vi "Alignment.vi"() -> ()   [LabVIEW 2010]
uses:
  <vilib>/Utility/inputDevices.llb/closeKeyboard.vi
  <vilib>/Utility/inputDevices.llb/keyboardAcquire.vi
panel:
  out "Q":bool
  out "Further":bool
  out "Nearer":bool
  out "End":bool=TRUE
  out "Right":bool
  out "Up":bool
  out "Left":bool
  out "Down":bool
  in  "Motor GPIB":u8=6 max=32 step=1 format="%#.0f"
  out "keys pressed":T1(array[ring])
  # "Press \"=\" for complete tower down."
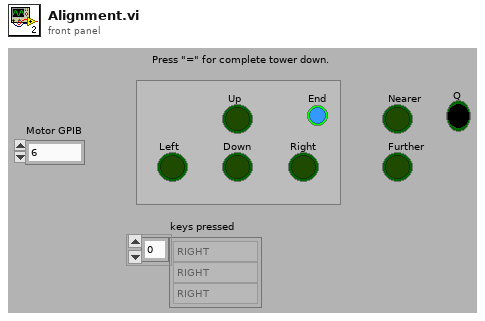
[diagram p1: front panel]
types:
  T1 = enum16{"0", "1", "2", "3", "4", "5", "6", "7", "8", "9", "A", "B", "C", "D", "E", "F", "G", "H", "I", "J", "K", "L", "M", "N", "O", "P", "Q", "R", "S", "T", "U", "V", "W", "X", "Y", "Z", "F1", "F2", "F3", "F4", "F5", "F6", "F7", "F8", "F9", "F10", "F11", "F12", "F13", "F14", "F15", "ADD", "BACK", "BACKSLASH", "CAPITAL", "COMMA", "DECIMAL", "DELETE", "DIVIDE", "DOWN", "END", "EQUALS", "ESCAPE", "GRAVE (`)", "HOME", "INSERT", "LBRACKET", "LCONTROL", "LEFT", "L ALT", "LSHIFT", "LWIN", "MINUS", "MULTIPLY", "NEXT", "NUMLOCK", "NUMPAD_0", "NUMPAD_1", "NUMPAD_2", "NUMPAD_3", "NUMPAD_4", "NUMPAD_5", "NUMPAD_6", "NUMPAD_7", "NUMPAD_8", "NUMPAD_9", "PAUSE", "PERIOD", "PRIOR (PG UP)", "RBRACKET", "RCONTROL", "RETURN", "RIGHT", "R ALT", "RSHIFT", "RWIN", "SCROLL", "SEMICOLON", "SLASH", "SPACE", "SUBTRACT", "TAB", "UP", "ENTER (num pad)", "' (quote)"}[]
  T2 = enum16{"0", "1", "2", "3", "4", "5", "6", "7", "8", "9", "A", "B", "C", "D", "E", "F", "G", "H", "I", "J", "K", "L", "M", "N", "O", "P", "Q", "R", "S", "T", "U", "V", "W", "X", "Y", "Z", "F1", "F2", "F3", "F4", "F5", "F6", "F7", "F8", "F9", "F10", "F11", "F12", "F13", "F14", "F15", "ADD", "BACK", "BACKSLASH", "CAPITAL", "COMMA", "DECIMAL", "DELETE", "DIVIDE", "DOWN", "END", "EQUALS", "ESCAPE", "GRAVE (`)", "HOME", "INSERT", "LBRACKET", "LCONTROL", "LEFT", "L ALT", "LSHIFT", "LWIN", "MINUS", "MULTIPLY", "NEXT", "NUMLOCK", "NUMPAD_0", "NUMPAD_1", "NUMPAD_2", "NUMPAD_3", "NUMPAD_4", "NUMPAD_5", "NUMPAD_6", "NUMPAD_7", "NUMPAD_8", "NUMPAD_9", "PAUSE", "PERIOD", "PRIOR (PG UP)", "RBRACKET", "RCONTROL", "RETURN", "RIGHT", "R ALT", "RSHIFT", "RWIN", "SCROLL", "SEMICOLON", "SLASH", "SPACE", "SUBTRACT", "TAB", "UP", "ENTER (num pad)", "' (quote)"}
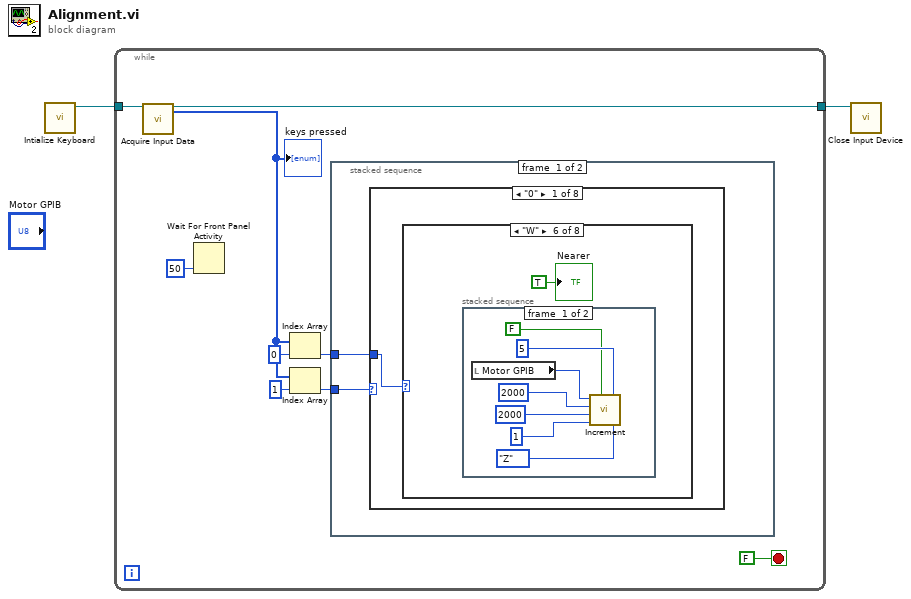
[diagram p0: block diagram]
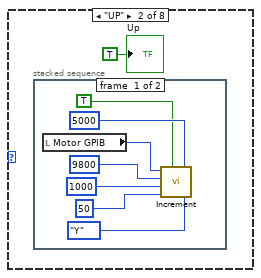
[diagram p3: hidden frame]
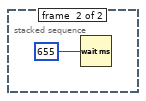
[diagram p4: hidden frame]
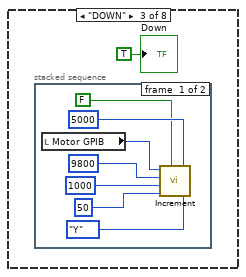
[diagram p5: hidden frame]
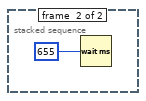
[diagram p6: hidden frame]
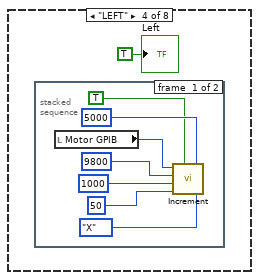
[diagram p7: hidden frame]
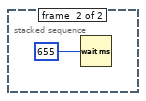
[diagram p8: hidden frame]
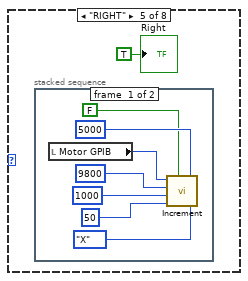
[diagram p9: hidden frame]
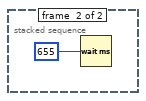
[diagram p10: hidden frame]
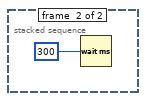
[diagram p11: hidden frame]
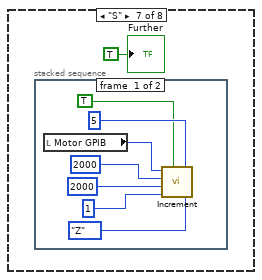
[diagram p12: hidden frame]
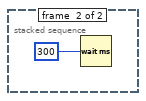
[diagram p13: hidden frame]
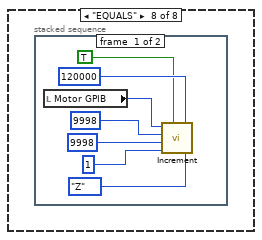
[diagram p14: hidden frame]
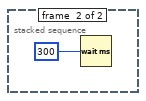
[diagram p15: hidden frame]
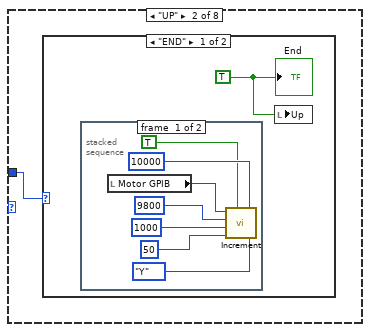
[diagram p16: hidden frame]
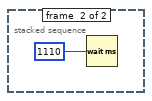
[diagram p17: hidden frame]
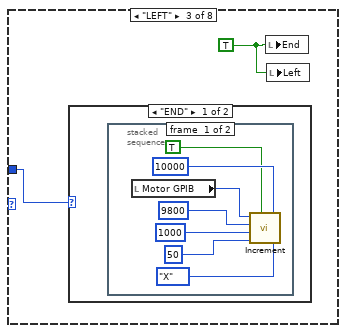
[diagram p19: hidden frame]
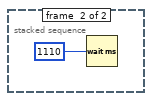
[diagram p20: hidden frame]
diagram:
  n1 = call <vilib>:"Intialize Keyboard.vi"() -> ("device ID"=w1:refnum<k1>)  [unwired: 10 in, 1 out]
  n2 = while {
    tunnel: w1 -> [w11]
    tunnel: [w10] -> w2
    stop <- FALSE stop-if-true
    n3 = call-poly <vilib>:"Acquire Input Data.vi"("device ID"=w11) -> ("device ID"=w10:refnum<k1>, "keys pressed"=w8:T1)  [unwired: 16 in, 1 out]
    "keys pressed" <- w8
    n4 = Wait For Front Panel Activity(1:50 ("timeout ms (-1 never timeout)")) -> ()  [unwired: 2 in, 1 out]
    n5 = Index Array(array=w8, index=0) -> (element=w4:T2)
    n6 = Index Array(array=w8, index=1) -> (element=w5:T2)
    n7 = stacked-sequence {
      tunnel: w5 -> [w13 _]
      tunnel: w4 -> [w12 _]
      frame #0 {
        n8 = case shown="\"0\"" w13 {
          tunnel: w12 -> [w14 w77 w87 w98 w107 w117 w127 _]
          frame "0" {
            n9 = case shown="\"W\"" w14 {
              frame "0", Default {
              }
              frame "UP" {
                n10 = stacked-sequence {
                  frame #0 {
                    n11 = local read "Motor GPIB"() -> (w22:u8)
                    n12 = call "Increment.vi"("GPIB_Addr"=w22, "F Speed"=u16 9800, "L Speed"=u16 1000, "Rate"=u16 50, "CCW 3"=TRUE, "Distance"=u32 5000, "Axis"=enum16{"X", "Y", "Z", "U", "V", "W"}."Y") -> ()
                  }
                  frame #1 {
                    n13 = Wait (ms)(milliseconds to wait=655 ("timeout ms (-1 never timeout)")) -> ()  [unwired: 1 out]
                  }
                }
                "Up" <- TRUE ("Up")
              }
              frame "DOWN" {
                n14 = stacked-sequence {
                  frame #0 {
                    n15 = local read "Motor GPIB"() -> (w31:u8)
                    n16 = call "Increment.vi"("GPIB_Addr"=w31, "F Speed"=u16 9800, "L Speed"=u16 1000, "Rate"=u16 50, "CCW 3"=FALSE, "Distance"=u32 5000, "Axis"=enum16{"X", "Y", "Z", "U", "V", "W"}."Y") -> ()
                  }
                  frame #1 {
                    n17 = Wait (ms)(milliseconds to wait=655 ("timeout ms (-1 never timeout)")) -> ()  [unwired: 1 out]
                  }
                }
                "Down" <- TRUE ("Down")
              }
              frame "LEFT" {
                n18 = stacked-sequence {
                  frame #0 {
                    n19 = local read "Motor GPIB"() -> (w40:u8)
                    n20 = call "Increment.vi"("GPIB_Addr"=w40, "F Speed"=u16 9800, "L Speed"=u16 1000, "Rate"=u16 50, "CCW 3"=TRUE, "Distance"=u32 5000, "Axis"=enum16{"X", "Y", "Z", "U", "V", "W"}."X") -> ()
                  }
                  frame #1 {
                    n21 = Wait (ms)(milliseconds to wait=655 ("timeout ms (-1 never timeout)")) -> ()  [unwired: 1 out]
                  }
                }
                "Left" <- TRUE ("Left")
              }
              frame "RIGHT" {
                n22 = stacked-sequence {
                  frame #0 {
                    n23 = local read "Motor GPIB"() -> (w49:u8)
                    n24 = call "Increment.vi"("GPIB_Addr"=w49, "F Speed"=u16 9800, "L Speed"=u16 1000, "Rate"=u16 50, "CCW 3"=FALSE, "Distance"=u32 5000, "Axis"=enum16{"X", "Y", "Z", "U", "V", "W"}."X") -> ()
                  }
                  frame #1 {
                    n25 = Wait (ms)(milliseconds to wait=655 ("timeout ms (-1 never timeout)")) -> ()  [unwired: 1 out]
                  }
                }
                "Right" <- TRUE ("Right")
              }
              frame "W" {
                n26 = stacked-sequence {
                  frame #0 {
                    n27 = local read "Motor GPIB"() -> (w58:u8)
                    n28 = call "Increment.vi"("GPIB_Addr"=w58, "F Speed"=u16 2000, "L Speed"=u16 2000, "Rate"=u16 1, "CCW 3"=FALSE, "Distance"=u32 5, "Axis"=enum16{"X", "Y", "Z", "U", "V", "W"}."Z") -> ()
                  }
                  frame #1 {
                    n29 = Wait (ms)(milliseconds to wait=300 ("timeout ms (-1 never timeout)")) -> ()  [unwired: 1 out]
                  }
                }
                "Nearer" <- TRUE ("Up")
              }
              frame "S" {
                n30 = stacked-sequence {
                  frame #0 {
                    n31 = local read "Motor GPIB"() -> (w67:u8)
                    n32 = call "Increment.vi"("GPIB_Addr"=w67, "F Speed"=u16 2000, "L Speed"=u16 2000, "Rate"=u16 1, "CCW 3"=TRUE, "Distance"=u32 5, "Axis"=enum16{"X", "Y", "Z", "U", "V", "W"}."Z") -> ()
                  }
                  frame #1 {
                    n33 = Wait (ms)(milliseconds to wait=300 ("timeout ms (-1 never timeout)")) -> ()  [unwired: 1 out]
                  }
                }
                "Further" <- TRUE ("Up")
              }
              frame "EQUALS" {
                n34 = stacked-sequence {
                  frame #0 {
                    n35 = local read "Motor GPIB"() -> (w75:u8)
                    n36 = call "Increment.vi"("GPIB_Addr"=w75, "F Speed"=u16 9998, "L Speed"=u16 9998, "Rate"=u16 1, "CCW 3"=TRUE, "Distance"=u32 120000, "Axis"=enum16{"X", "Y", "Z", "U", "V", "W"}."Z") -> ()
                  }
                  frame #1 {
                    n37 = Wait (ms)(milliseconds to wait=300 ("timeout ms (-1 never timeout)")) -> ()  [unwired: 1 out]
                  }
                }
              }
            }
          }
          frame "UP" {
            n38 = case shown="\"END\"" w77 {
              frame "END" {
                w78 = TRUE ("RCtrl")
                n39 = stacked-sequence {
                  frame #0 {
                    n40 = local read "Motor GPIB"() -> (w85:u8)
                    n41 = call "Increment.vi"("GPIB_Addr"=w85, "F Speed"=u16 9800, "L Speed"=u16 1000, "Rate"=u16 50, "CCW 3"=TRUE, "Distance"=u32 10000, "Axis"=enum16{"X", "Y", "Z", "U", "V", "W"}."Y") -> ()
                  }
                  frame #1 {
                    n42 = Wait (ms)(milliseconds to wait=1110 ("timeout ms (-1 never timeout)")) -> ()  [unwired: 1 out]
                  }
                }
                n43 = local write "Up"(w78) -> ()
                "End" <- w78
              }
              frame "2", Default {
              }
            }
          }
          frame "LEFT" {
            w88 = TRUE ("CCW 3")
            n44 = case shown="\"END\"" w87 {
              frame "END" {
                n45 = stacked-sequence {
                  frame #0 {
                    n46 = local read "Motor GPIB"() -> (w95:u8)
                    n47 = call "Increment.vi"("GPIB_Addr"=w95, "F Speed"=u16 9800, "L Speed"=u16 1000, "Rate"=u16 50, "CCW 3"=TRUE, "Distance"=u32 10000, "Axis"=enum16{"X", "Y", "Z", "U", "V", "W"}."X") -> ()
                  }
                  frame #1 {
                    n48 = Wait (ms)(milliseconds to wait=1110 ("timeout ms (-1 never timeout)")) -> ()  [unwired: 1 out]
                  }
                }
              }
              frame "2", Default {
              }
            }
            n49 = local write "End"(w88) -> ()
            n50 = local write "Left"(w88) -> ()
          }
          frame "RIGHT" {
            w97 = TRUE ("CCW 3")
            n51 = case shown="\"END\"" w98 {
              frame "END" {
                n52 = stacked-sequence {
                  frame #0 {
                    n53 = local read "Motor GPIB"() -> (w105:u8)
                    n54 = call "Increment.vi"("GPIB_Addr"=w105, "F Speed"=u16 9800, "L Speed"=u16 1000, "Rate"=u16 50, "CCW 3"=FALSE, "Distance"=u32 10000, "Axis"=enum16{"X", "Y", "Z", "U", "V", "W"}."X") -> ()
                  }
                  frame #1 {
                    n55 = Wait (ms)(milliseconds to wait=1110 ("timeout ms (-1 never timeout)")) -> ()  [unwired: 1 out]
                  }
                }
              }
              frame "2", Default {
              }
            }
            n56 = local write "Right"(w97) -> ()
            n57 = local write "End"(w97) -> ()
          }
          frame "END" {
            n58 = case shown="\"DOWN\"" w107 {
              frame "0", Default {
              }
              frame "DOWN" {
                w108 = TRUE ("Ctrl")
                n59 = stacked-sequence {
                  frame #0 {
                    n60 = local read "Motor GPIB"() -> (w115:u8)
                    n61 = call "Increment.vi"("GPIB_Addr"=w115, "F Speed"=u16 9800, "L Speed"=u16 1000, "Rate"=u16 50, "CCW 3"=FALSE, "Distance"=u32 10000, "Axis"=enum16{"X", "Y", "Z", "U", "V", "W"}."Y") -> ()
                  }
                  frame #1 {
                    n62 = Wait (ms)(milliseconds to wait=1110 ("timeout ms (-1 never timeout)")) -> ()  [unwired: 1 out]
                  }
                }
                n63 = local write "End"(w108) -> ()
                n64 = local write "Down"(w108) -> ()
              }
            }
          }
          frame "W" {
            n65 = case shown="\"E\"" w117 {
              frame "7", Default {
              }
              frame "E" {
                w118 = TRUE ("Up")
                n66 = stacked-sequence {
                  frame #0 {
                    n67 = local read "Motor GPIB"() -> (w125:u8)
                    n68 = call "Increment.vi"("GPIB_Addr"=w125, "F Speed"=u16 9999, "L Speed"=u16 9999, "Rate"=u16 1, "CCW 3"=FALSE, "Distance"=u32 3000, "Axis"=enum16{"X", "Y", "Z", "U", "V", "W"}."Z") -> ()
                  }
                  frame #1 {
                    n69 = Wait (ms)(milliseconds to wait=300 ("timeout ms (-1 never timeout)")) -> ()  [unwired: 1 out]
                  }
                }
                n70 = local write "Nearer"(w118) -> ()
                "Q" <- w118
              }
            }
          }
          frame "S" {
            n71 = case shown="\"E\"" w127 {
              frame "7", Default {
              }
              frame "E" {
                w128 = TRUE ("Up")
                n72 = stacked-sequence {
                  frame #0 {
                    n73 = local read "Motor GPIB"() -> (w135:u8)
                    n74 = call "Increment.vi"("GPIB_Addr"=w135, "F Speed"=u16 9999, "L Speed"=u16 9999, "Rate"=u16 1, "CCW 3"=TRUE, "Distance"=u32 3000, "Axis"=enum16{"X", "Y", "Z", "U", "V", "W"}."Z") -> ()
                  }
                  frame #1 {
                    n75 = Wait (ms)(milliseconds to wait=300 ("timeout ms (-1 never timeout)")) -> ()  [unwired: 1 out]
                  }
                }
                n76 = local write "Further"(w128) -> ()
                n77 = local write "Q"(w128) -> ()
              }
            }
          }
          frame "2", Default {
          }
        }
      }
      frame #1 {
        w137 = FALSE ("Up")
        n78 = local write "Up"(w137) -> ()
        n79 = local write "Down"(w137) -> ()
        n80 = local write "Left"(w137) -> ()
        n81 = local write "Right"(w137) -> ()
        n82 = local write "End"(w137) -> ()
        n83 = local write "Further"(w137) -> ()
        n84 = local write "Nearer"(w137) -> ()
        n85 = local write "Q"(w137) -> ()
      }
    }
  }
  n86 = call-poly <vilib>:"Close Input Device.vi"("device ID"=w2) -> ()  [unwired: 9 in, 1 out]
